vi "Aero_Chilled_Water_PID.vi"(1 "Tweak in working section demanded temp":dbl, 2 "Tunnel Speed":dbl, 3 "Present Value":dbl=15.0 format="%.2f", 4 "Reset PID":bool, 5 "Current Time":dbl, 6 "Setpoint":dbl=15.0 format="%.2f") -> (0 "Dem Output":dbl format="%.2f")   [LabVIEW 2022 SP3]
uses:
  <vilib>/Analysis/NI_AALPro.lvlib
panel:
  out "Speed Factor 0 to 1":dbl
  out "Derivative":dbl(graph)
  out "Integral":dbl(graph)
  out "Proportional":dbl(graph)
  out "Error":dbl(graph)
  in  "O/P deadband":dbl format="%.2f"
  in  "Kp Deadband":dbl format="%.2f"
  in  "Derivative History":i32=60
  out "deadbanded error":dbl format="%.2f"
  in  "P":bool=TRUE
  in  "D":bool=TRUE
  in  "I":bool=TRUE
  in  "Manual Demand":dbl min=0.0 max=100.0 format="%.2f"
  in  "Manual Override":bool
  out "Control Sum":dbl format="%.2f"
  out "error differential":dbl format="%.5f"
  in  "Kd":dbl=1600.0 format="%.2f"
  in  "Ki":dbl=0.15 format="%.2f"
  in  "Kp":dbl=15.0 format="%.2f"
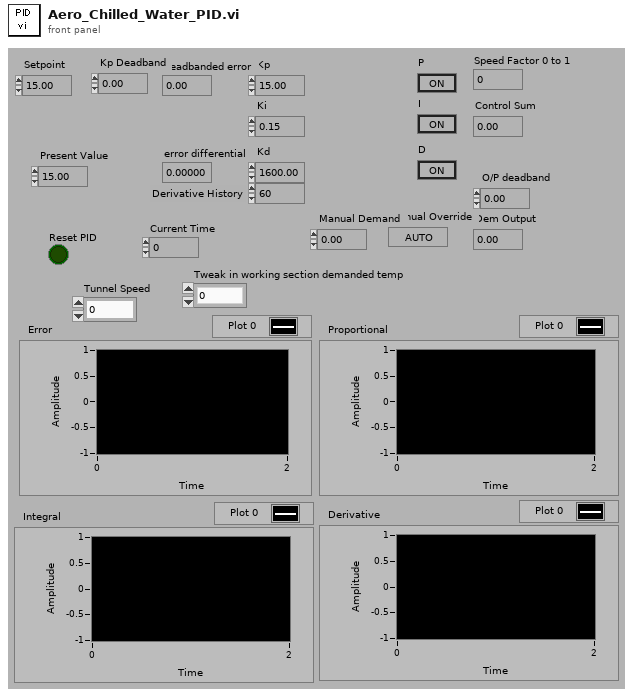
[diagram p1: front panel]
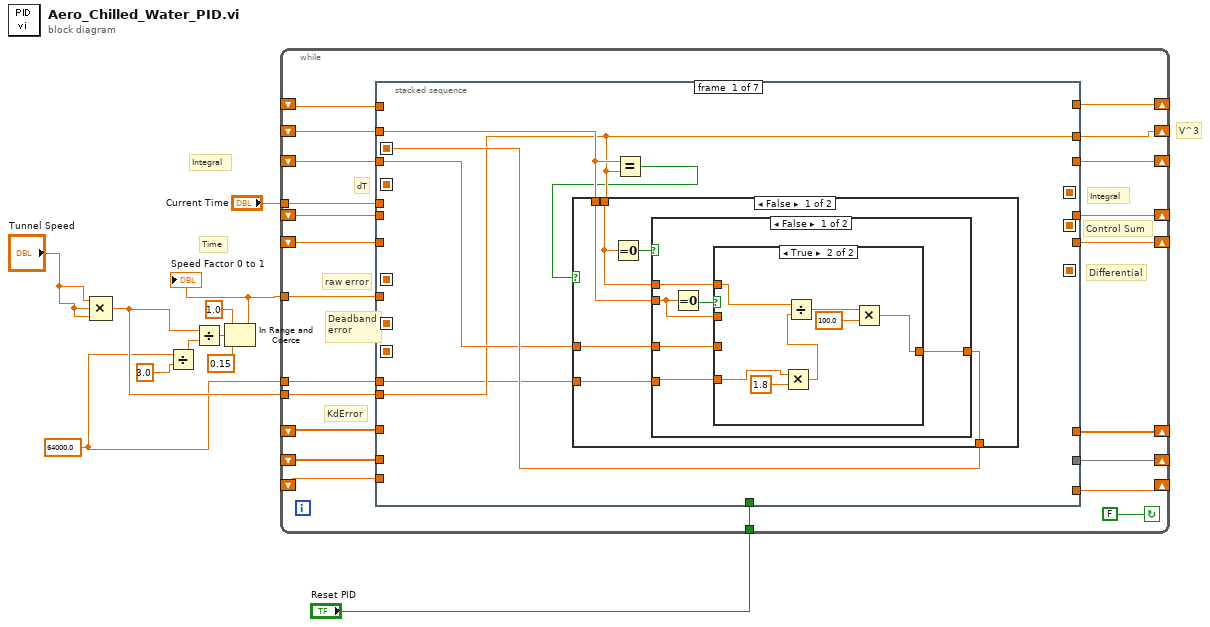
[diagram p0: block diagram]
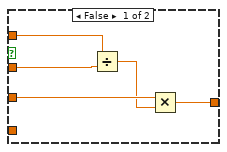
[diagram p2: hidden frame]
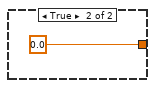
[diagram p3: hidden frame]
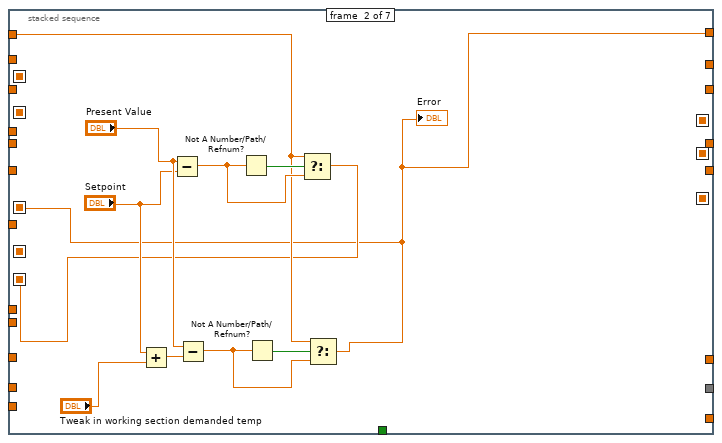
[diagram p5: hidden frame]
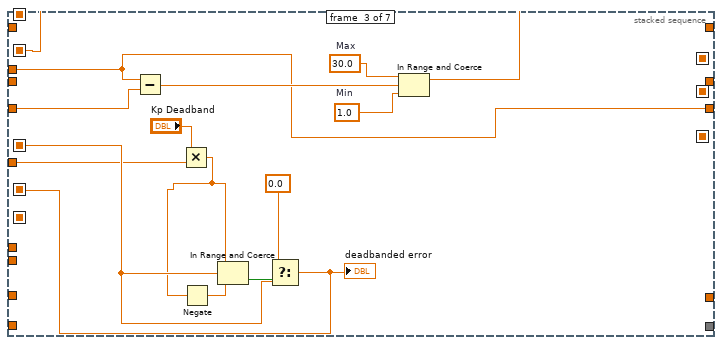
[diagram p6: hidden frame]
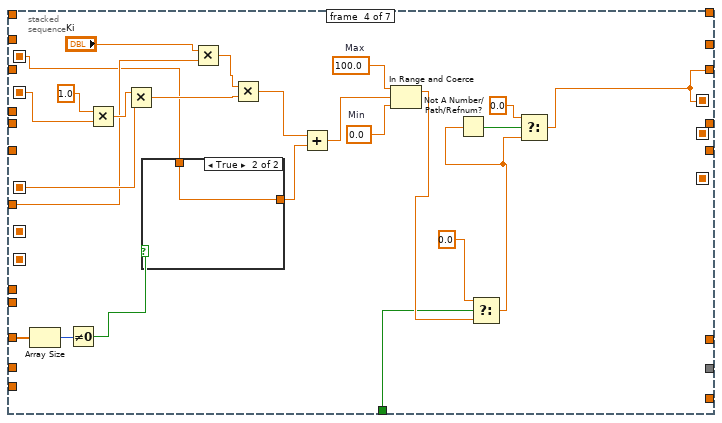
[diagram p7: hidden frame]
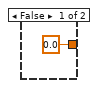
[diagram p8: hidden frame]
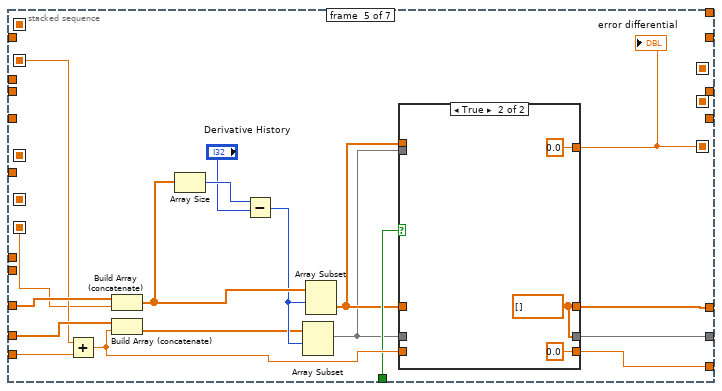
[diagram p9: hidden frame]
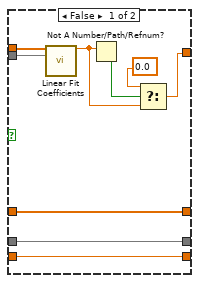
[diagram p10: hidden frame]
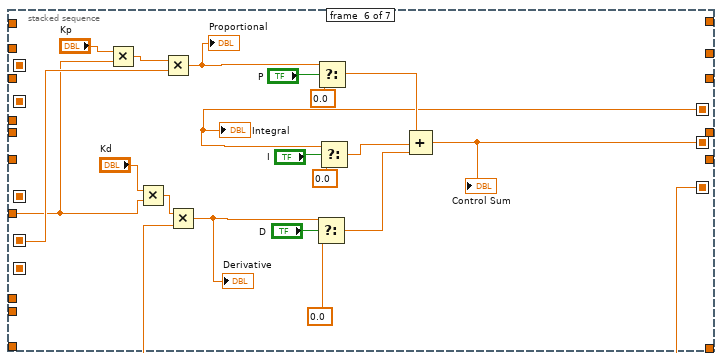
[diagram p11: hidden frame]
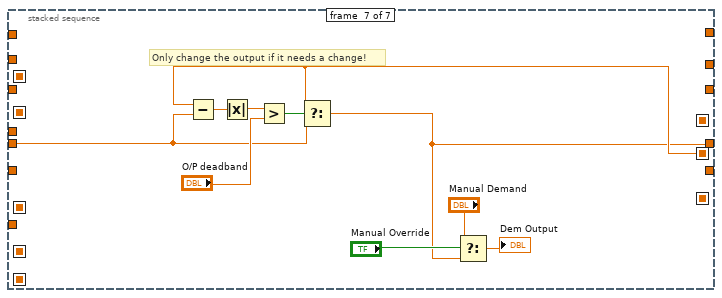
[diagram p12: hidden frame]
diagram:
  w7 = 64000.0
  # "V^3"
  # "Integral"
  # "Time"
  n1 = Compound Arithmetic op=MULTIPLY("Tunnel Speed", "Tunnel Speed", "Tunnel Speed") -> (w8:dbl)
  n2 = Divide(x=w7, y=3.0) -> (x/y=w5:dbl)
  n3 = Divide(x=w8, y=w5) -> (x/y=w4:dbl)
  n4 = In Range and Coerce(upper limit=1.0, x=w4, lower limit=0.15) -> (coerced(x)=w1:dbl)  [unwired: 1 out]
  "Speed Factor 0 to 1" <- w1
  n5 = while {
    shift-left: _ -> [w20]
    shift-right: [w19] -> _
    shift-left: _ -> [w22]
    shift-right: [w21] -> _
    shift-left: _ -> [w24]
    shift-right: [w23] -> _
    tunnel: "Current Time" -> [w29]
    shift-left: _ -> [w26]
    shift-right: [w25] -> _
    shift-left: _ -> [w28]
    shift-right: [w27] -> _
    shift-left: _ -> [w30]
    shift-right: [w31] -> _
    shift-left: _ -> [w33]
    shift-right: [w32] -> _
    tunnel: "Reset PID" -> [w17]
    tunnel: w1 -> [w16]
    tunnel: w8 -> [w15]
    shift-right: [w14] -> _
    shift-left: _ -> [w13]
    tunnel: w7 -> [w12]
    stop <- FALSE continue-if-true
    # "KdError"
    # "Control Sum"
    # "raw error"
    # "Differential"
    # "Integral"
    # "Deadband\nerror"
    # "dT"
    n6 = stacked-sequence {
      seq-local: [_ _ w80 _ _ _ _] -> [_ _ _ w104 w126 _ _]
      seq-local: [_ _ w88 _ _ _ _] -> [_ _ _ _ _ w156 _]
      seq-local: [_ _ _ _ w127 _ _] -> [_ _ _ _ _ w155 _]
      seq-local: [_ _ _ w98 _ _ _] -> [_ _ _ _ _ w152 _]
      seq-local: [_ w66 _ _ _ _ _] -> [_ _ w81 w112 _ _ _]
      seq-local: [_ _ _ _ _ w157 _] -> [_ _ _ _ _ _ w170]
      seq-local: [_ w67 _ _ _ _ _] -> [_ _ _ _ w124 _ _]
      seq-local: [w39 _ _ _ _ _ _] -> [_ _ _ w91 _ _ _]
      tunnel: w33 -> [_ _ w85 _ _ _ _]
      tunnel: [_ _ w83 _ _ _ _] -> w32
      tunnel: [_ _ _ w98 _ _ _] -> w31
      tunnel: w30 -> [w38 _ _ _ _ _ _]
      tunnel: w29 -> [_ _ w83 _ _ _ _]
      tunnel: w28 -> [_ _ _ w111 w134 _ _]
      tunnel: [_ _ _ _ w120 _ _] -> w27
      tunnel: w26 -> [_ _ _ _ w133 _ _]
      tunnel: [_ _ _ _ w118 _ _] -> w25
      tunnel: w24 -> [_ _ _ _ _ _ w168]
      tunnel: [_ _ _ _ _ _ w167] -> w23
      tunnel: w22 -> [_ _ _ _ w125 _ _]
      tunnel: [_ _ _ _ w123 _ _] -> w21
      tunnel: w20 -> [_ w72 _ _ _ _ _]
      tunnel: [_ w66 _ _ _ _ _] -> w19
      tunnel: w17 -> [_ _ _ w99 w121 _ _]
      tunnel: w16 -> [_ _ w77 w92 _ w148 _]
      tunnel: w15 -> [w36 _ _ _ _ _ _]
      tunnel: [w36 _ _ _ _ _ _] -> w14
      tunnel: w13 -> [w37 _ _ _ _ _ _]
      tunnel: w12 -> [w34 _ _ _ _ _ _]
      frame #0 {
        n7 = Equal?(x=w37, y=w36) -> (x = y?=w35:bool)
        n8 = case shown="False" w35 {
          tunnel: w36 -> [w42 _]
          tunnel: w37 -> [w45 _]
          tunnel: [w43 w65] -> w39
          tunnel: w38 -> [w44 w65]
          tunnel: w34 -> [w40 _]
          frame False {
            n9 = Equal To 0?(x=w42) -> (x = 0?=w41:bool)
            n10 = case shown="False" w41 {
              tunnel: w45 -> [w46 _]
              tunnel: w44 -> [w51 _]
              tunnel: [w50 0.0] -> w43
              tunnel: w42 -> [w49 _]
              tunnel: w40 -> [w48 _]
              frame False {
                n11 = Equal To 0?(x=w46) -> (x = 0?=w47:bool)
                n12 = case shown="True" w47 {
                  tunnel: w51 -> [w56 _]
                  tunnel: [w54 w57] -> w50
                  tunnel: w49 -> [w53 w61]
                  tunnel: w48 -> [_ w62]
                  tunnel: w46 -> [w52 _]
                  frame False {
                    n13 = Divide(x=w53, y=w52) -> (x/y=w55:dbl)
                    n14 = Multiply(x=w56, y=w55) -> (x*y=w54:dbl)
                  }
                  frame True {
                    n15 = Multiply(x=w62, y=1.8) -> (x*y=w60:dbl)
                    n16 = Divide(x=w61, y=w60) -> (x/y=w59:dbl)
                    n17 = Multiply(x=w59, y=100.0) -> (x*y=w57:dbl)
                  }
                }
              }
              frame True {
              }
            }
          }
          frame True {
          }
        }
      }
      frame #1 {
        n18 = Add(x="Setpoint", y="Tweak in working section demanded temp") -> (x+y=w68:dbl)
        n19 = Subtract(x="Present Value", y="Setpoint") -> (x-y=w75:dbl)
        n20 = Subtract(x="Present Value", y=w68) -> (x-y=w74:dbl)
        n21 = Not A Number/Path/Refnum?(number/path/refnum=w75) -> (NaN/Path/Refnum?=w76:bool)
        n22 = Not A Number/Path/Refnum?(number/path/refnum=w74) -> (NaN/Path/Refnum?=w73:bool)
        n23 = Select(t=w72, s=w76, f=w75) -> (s? t:f=w67:dbl)
        n24 = Select(t=w72, s=w73, f=w74) -> (s? t:f=w66:dbl)
        "Error" <- w66
      }
      frame #2 {
        w86 = 1.0  # Min
        w87 = 30.0  # Max
        n25 = Subtract(x=w83, y=w85) -> (x-y=w84:dbl)
        n26 = Multiply(x="Kp Deadband", y=w77) -> (x*y=w78:dbl)
        n27 = Negate(x=w78) -> (-x=w82:dbl)
        n28 = In Range and Coerce(upper limit=w78, x=w81, lower limit=w82) -> (In Range?=w89:bool)  [unwired: 1 out]
        n29 = Select(t=0.0, s=w89, f=w81) -> (s? t:f=w88:dbl)
        "deadbanded error" <- w88
        n30 = In Range and Coerce(upper limit=w87, x=w84, lower limit=w86) -> (coerced(x)=w80:dbl)  [unwired: 1 out]
      }
      frame #3 {
        w114 = 0.0  # Min
        w97 = 100.0  # Max
        n31 = Array Size(array=w111) -> (size(s)=w110:i32)
        n32 = Not Equal To 0?(x=w110) -> (x != 0?=w109:bool)
        n33 = Multiply(x=1.0, y=w104) -> (x*y=w103:dbl)
        n34 = Multiply(x=w103, y=w112) -> (x*y=w96:dbl)
        n35 = case shown="True" w109 {
          tunnel: [0.0 ("Min") w116] -> w108
          tunnel: w91 -> [_ w116]
          frame False {
          }
          frame True {
          }
        }
        n36 = Multiply(x="Ki", y=w92) -> (x*y=w93:dbl)
        n37 = Multiply(x=w93, y=w96) -> (x*y=w95:dbl)
        n38 = Add(x=w95, y=w108) -> (x+y=w113:dbl)
        n39 = In Range and Coerce(upper limit=w97, x=w113, lower limit=w114) -> (coerced(x)=w101:dbl)  [unwired: 1 out]
        n40 = Select(t=0.0, s=w99, f=w101) -> (s? t:f=w100:dbl)
        n41 = Not A Number/Path/Refnum?(number/path/refnum=w100) -> (NaN/Path/Refnum?=w106:bool)
        n42 = Select(t=0.0, s=w106, f=w100) -> (s? t:f=w98:dbl)
      }
      frame #4 {
        n43 = Add(x=w126, y=w125) -> (x+y=w122:dbl)
        n44 = Build Array (concatenate)(w134, w124) -> (w130:dbl[])
        n45 = Build Array (concatenate)(w133, w122) -> (w128:dbl[])
        n46 = Array Size(array=w130) -> (size(s)=w132:i32)
        n47 = Subtract(x=w132, y="Derivative History") -> (x-y=w129:i32)
        n48 = Array Subset(array=w128, index=w129) -> (w117:dbl[])  [unwired: 1 in]
        n49 = Array Subset(array=w130, index=w129) -> (w119:dbl[])  [unwired: 1 in]
        n50 = case shown="True" w121 {
          tunnel: w119 -> [w143 _]
          tunnel: [w137 0.0 ("slope")] -> w127
          tunnel: w117 -> [w142 _]
          tunnel: [w138 0.0] -> w123
          tunnel: w122 -> [w138 _]
          tunnel: [w136 w145] -> w120
          tunnel: w119 -> [w136 _]
          tunnel: [w135 w145] -> w118
          tunnel: w117 -> [w135 _]
          frame False {
            n51 = call <vilib>:"Linear Fit Coefficients.vi"("Y"=w143, "X"=w142) -> ("slope"=w139:dbl)  [unwired: 3 in, 10 out]
            n52 = Not A Number/Path/Refnum?(number/path/refnum=w139) -> (NaN/Path/Refnum?=w141:bool)
            n53 = Select(t=0.0 ("f"), s=w141, f=w139) -> (s? t:f=w137:dbl)
          }
          frame True {
            w145 = dbl[] []
          }
        }
        "error differential" <- w127
      }
      frame #5 {
        n54 = Multiply(x="Kp", y=w148) -> (x*y=w147:dbl)
        n55 = Multiply(x="Kd", y=w148) -> (x*y=w150:dbl)
        n56 = Multiply(x=w147, y=w156) -> (x*y=w153:dbl)
        "Proportional" <- w153
        n57 = Multiply(x=w150, y=w155) -> (x*y=w154:dbl)
        "Derivative" <- w154
        n58 = Select(t=w154, s="D", f=0.0) -> (s? t:f=w159:dbl)
        n59 = Select(t=w153, s="P", f=0.0) -> (s? t:f=w165:dbl)
        n60 = Select(t=w152, s="I", f=0.0) -> (s? t:f=w158:dbl)
        n61 = Compound Arithmetic op=ADD(w165, w158, w159) -> (w157:dbl)
        "Control Sum" <- w157
        "Integral" <- w152
      }
      frame #6 {
        # "Only change the output if it needs a change!"
        n62 = Subtract(x=w170, y=w168) -> (x-y=w173:dbl)
        n63 = Absolute Value(x=w173) -> (abs(x)=w172:dbl)
        n64 = Greater?(x=w172, y="O/P deadband") -> (0:w171:bool)
        n65 = Select(t=w170, s=w171, f=w168) -> (s? t:f=w167:dbl)
        n66 = Select(t="Manual Demand", s="Manual Override", f=w167) -> (s? t:f=→"Dem Output":dbl)
      }
    }
  }
